vi "Config Display.vi"(0 "VISA resource name":refnum<visa-resource-name>, 1 "Number of Fields (1)":dbl=1.0 min=1.0 max=8.0 step=1.0, 3 "Backlight (T: Backlight On)":bool=TRUE, 4 "Output Display\nMode (0: Current)":u16(ring) items=["Current", "Power"], 5 "error in (no error)":errorcluster, 6 "Loop (0: 1)":u16(ring) items=["1", "2"], 7 "Display Contrast (50)":dbl=50.0 min=0.0 max=100.0 step=1.0, 8 "Source (0: Kelvin)":u16(ring) items=["Kelvin", "Celsius", "Sensor Units", "Linear Data", "Min Data", "Max Data"], 9 "Input (0: A)":u16(ring) items=["A", "B", "C", "D"], 10 "Heater Resistance (25)":dbl=25.0 min=1.0 max=1000.0 step=1.0, 11 "Large Output (F: Disable)":bool, 12 "Number of Loops (0: None)":u16(ring) items=["None", "Loop 1", "Loop 2", "Both Loops"], 13 "Field (1)":dbl=1.0 min=1.0 max=8.0 step=1.0) -> (14 "VISA resource name out":refnum<visa-resource-name>, 19 "error out":errorcluster)   [LabVIEW 2020, in "Lake Shore Cryotronics 340.lvlib"]
doc: "This VI Configures the parameters of the main display, the displayed field, and the control loop's display."
uses:
  Lake Shore Cryotronics 340.lvlib
panel:
  # "Main Display Pararmeters"
  # "Displayed Field Parameters"
  # "Backlight On\nBacklight Off"
  # "Enable\nDisable"
  # "Control Loop's Display Parameters"
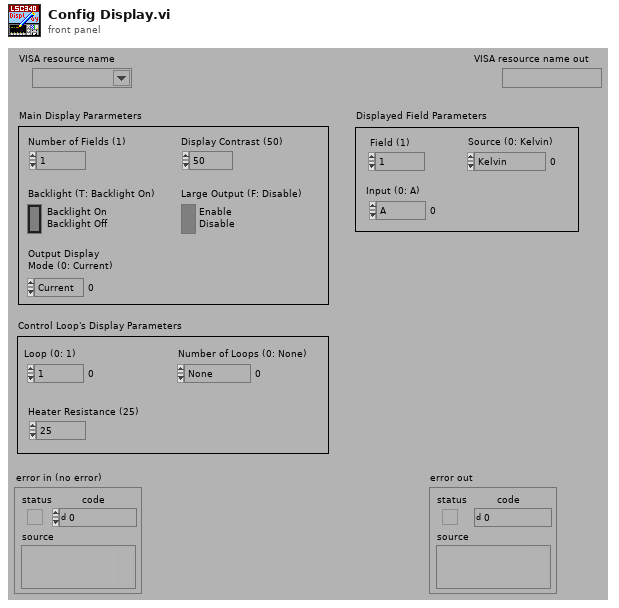
[diagram p1: front panel]
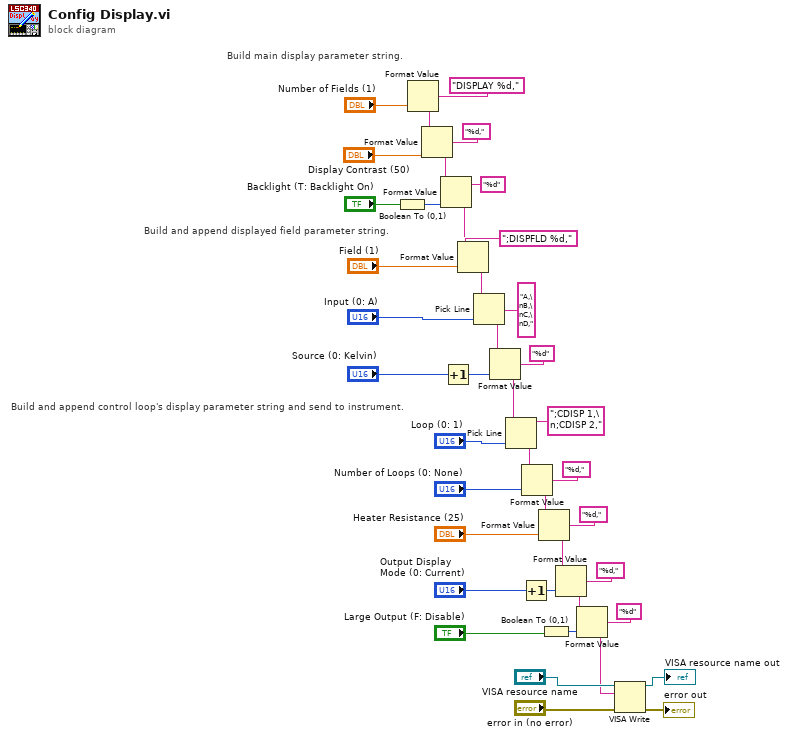
[diagram p0: block diagram]
diagram:
  # "Build and append control loop's display parameter string and send to instrument."
  # "Build and append displayed field parameter string."
  # "Build main display parameter string."
  n1 = Boolean To (0,1)(Boolean="Backlight (T: Backlight On)") -> (0, 1=w38:i16)
  n2 = Format Value(format string="DISPLAY %d,", value (0)="Number of Fields (1)") -> (output string=w37:string)  [unwired: 1 in]
  n3 = Format Value(string ("")=w37, format string="%d,", value (0)="Display Contrast (50)") -> (output string=w41:string)
  n4 = Format Value(string ("")=w41, format string="%d", value (0)=w38) -> (output string=w23:string)
  n5 = Increment(x="Source (0: Kelvin)") -> (x+1=w32:u16)
  n6 = Format Value(string ("")=w23, format string=";DISPFLD %d,", value (0)="Field (1)") -> (output string=w28:string)
  n7 = Pick Line(string ("")=w28, multi-line string="A,\nB,\nC,\nD,", line index="Input (0: A)") -> (output string=w31:string)
  n8 = Format Value(string ("")=w31, format string="%d", value (0)=w32) -> (output string=w1:string)
  n9 = Pick Line(string ("")=w1, multi-line string=";CDISP 1,\n;CDISP 2,", line index="Loop (0: 1)") -> (output string=w18:string)
  n10 = Increment(x="Output Display\nMode (0: Current)") -> (x+1=w7:u16)
  n11 = Format Value(string ("")=w18, format string="%d,", value (0)="Number of Loops (0: None)") -> (output string=w15:string)
  n12 = Format Value(string ("")=w15, format string="%d,", value (0)="Heater Resistance (25)") -> (output string=w12:string)
  n13 = Boolean To (0,1)(Boolean="Large Output (F: Disable)") -> (0, 1=w9:i16)
  n14 = Format Value(string ("")=w12, format string="%d,", value (0)=w7) -> (output string=w8:string)
  n15 = Format Value(string ("")=w8, format string="%d", value (0)=w9) -> (output string=w2:string)
  n16 = VISA Write(VISA resource name="VISA resource name", write buffer=w2, error in (no error)="error in (no error)") -> (VISA resource name out=→"VISA resource name out":refnum<visa-resource-name>, error out=→"error out":errorcluster)  [unwired: 1 out]
